vi "from seconds from midnight.vi"(11 "seconds from 00:00":dbl) -> (0 "hour":i32, 1 "minute":i32, 2 "second":i32, 3 "fractional second":dbl)   [LabVIEW 2020]
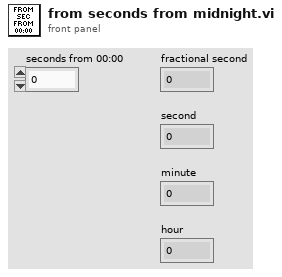
[diagram p1: front panel]
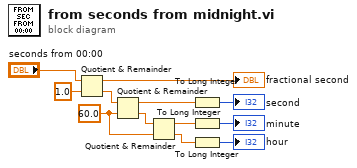
[diagram p0: block diagram]
diagram:
  w7 = 60.0 ("y")
  n1 = Quotient & Remainder(x="seconds from 00:00", y=1.0) -> (x-y*floor(x/y)=→"fractional second":dbl, floor(x/y)=w4:dbl)
  n2 = Quotient & Remainder(x=w4, y=w7) -> (x-y*floor(x/y)=w5:dbl, floor(x/y)=w6:dbl)
  n3 = Quotient & Remainder(x=w6, y=w7) -> (x-y*floor(x/y)=w8:dbl, floor(x/y)=w9:dbl)
  n4 = To Long Integer(number=w5) -> (32bit integer=→"second":i32)
  n5 = To Long Integer(number=w8) -> (32bit integer=→"minute":i32)
  n6 = To Long Integer(number=w9) -> (32bit integer=→"hour":i32)
